vi "Write Section - Double.vi"(6 "Create file if not found? (T)":bool=TRUE, 7 "Value":dbl, 8 "error in (no error)":errorcluster, 9 "key":string, 10 "section":string, 11 "Path":path) -> (0 "error out":errorcluster)   [LabVIEW 2019, in "TSC File IO.lvlib"]
doc: "This VI will write a section/cluster configuration file with type DBL.\n\nInputs:\n-Path [path] - a path to the file\n-section [string] - the section string in the configuration file\n-key [string] - the key to be read in the configuration file\n-value [DBL] - the output data written\n-error in\n\nOutputs:\n-error out\n_________________________________________________________________________\n<b>Code Developed By:</b>\nDaniel Coons\nTechnology Service Corporation\n1983 S Liberty Drive\nBloomington, IN 47403\nPhone: 812 558-7100\ndaniel.coons@tsc.com\nwww.tsc.com\n\n<b>Date Created:</b> 05 SEP 2014\n<b>Date Updated:</b> 13 APR 2020"
uses:
  TSC File IO.lvlib
  <vilib>/Utility/config.llb/NI_LVConfig.lvlib
  <vilib>/Utility/config.llb/Write Key (Double).vi
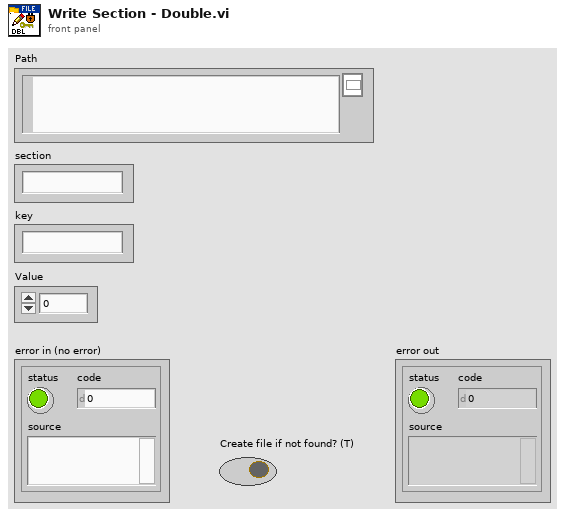
[diagram p1: front panel]
types:
  T1 = typedef "NI_LVConfig.lvlib/Config Data RefNum.ctl" = refnum<k1>
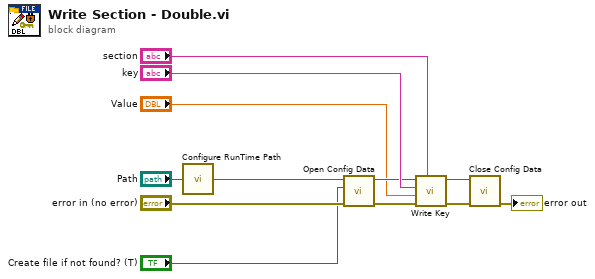
[diagram p0: block diagram]
diagram:
  n1 = call "Configure RunTime Path.vi"("Input Path"="Path") -> ("Updated Path"=w2:path)
  n2 = call <vilib>:"Open Config Data.vi"("error in (no error)"="error in (no error)", "create file if necessary (T)"="Create file if not found? (T)", "configuration file path"=w2) -> ("error out"=w5:errorcluster, "refnum"=w6:T1)  [unwired: 6 in, 1 out]
  n3 = call-poly <vilib>:"Write Key.vi"("section"="section", "error in (no error)"=w5, "value"="Value", "key"="key", "refnum"=w6) -> ("error out"=w7:errorcluster, "refnum out"=w8:T1)  [unwired: 4 in, 1 out]
  n4 = call <vilib>:"Close Config Data.vi"("error in (no error)"=w7, "refnum"=w8) -> ("error out"=→"error out":errorcluster)  [unwired: 8 in, 1 out]
